vi "fpga_main.vi"() -> ()   [LabVIEW 2025]
uses:
  <vilib>/rvi/Emulation/niFpgaGetClockAttributes.vi
  <vilib>/rvi/Emulation/niFpgaSctlEmulationGetInTimedLoop.vi
  <vilib>/rvi/Emulation/niFpgaEmulationReportErrorSimple.vi
  <vilib>/rvi/Emulation/niFpgaEmulationIsFPGAContextNoSignature.vi
  <vilib>/rvi/errors/niFpgaSetErrorForExecOnDevCompSimple.vi
  <vilib>/rvi/eio/common/nirviEmuReportErrorAndStop.vi
  <vilib>/rvi/DataTransferAndStorage/Container/Common/niFpgaContainerGetUniqueNameForEmu.vi
  <vilib>/rvi/FIFO/Fifo_Resource/nirvififoEmulationSetSize.vi
  <vilib>/rvi/FIFO/Fifo_Resource/nirviFifoEmulationQueueMgr.vi
  <instcachedir>/0/nirviFifoEmulationQueueMgr_E5CAEC123FF24DC58D834DCA3CDAA9B5.lvgen/nirviFifoEmulationQueueMgr_E5CAEC123FF24DC58D834DCA3CDAA9B5_001.vi
  <vilib>/Utility/error.llb/Clear Errors.vi
  <vilib>/rvi/FIFO/Fifo_Resource/nirvififoEmulationCreateLock.vi
  <vilib>/rvi/Emulation/niFpgaProcessEmulError.vi
  <vilib>/rvi/FIFO/Fifo_Resource/nirvififoEmulationObtainLock.vi
  <vilib>/rvi/FIFO/Fifo_Resource/nirvififoEmulationReleaseLock.vi
  <vilib>/rvi/occurrence/nirviWaitOnOccurrenceBase.vi
  <vilib>/rvi/errors/nirviReportUnexpectedCaseInternalError.vi
  <vilib>/rvi/errors/nirviReportUnexpectedCaseInternalError (U32).vi
  <vilib>/eio/utilities/niEioResolveVilibRelativePath.vi
  <vilib>/rvi/interface/RandomDataEmulation/niFpgaRandomDataHandleErrors.vi
  <vilib>/rvi/Emulation/niFpgaCriticalErrorInLSC.vi
  <vilib>/rvi/eio/common/nirviEmuTemplateMethod_errors.vi
  <vilib>/rvi/Memory/Memory_Emulation/nirvimemoryFastEmulation.vi
  <vilib>/rvi/Memory/Memory_Emulation/nirvimemoryEmulation.vi
  <vilib>/rvi/FIFO/Fifo_Resource/nirvififoEmulationDetermineInputValidOut.vi
  <vilib>/rvi/DataTransferAndStorage/Container/XNode/niFpgaContainer.xnode
  <vilib>/rvi/FIFO/Fifo_Resource/nirvififoEmulationRead.vi
  <vilib>/rvi/interface/RandomDataEmulation/nirviRandomDataFpgaReadWriteTemplate.vi
  <vilib>/eio/EIONode/EIONode.xnode
  <vilib>/rvi/FIFO/Fifo_Resource/nirvififoEmulationWrite.vi
panel:
  in  "Var data":cluster{"Placeholder":i16, "Trigger":bool}
  in  "Time delay_Send":u16=1250
  in  "Time Delay_Read":u16=1250
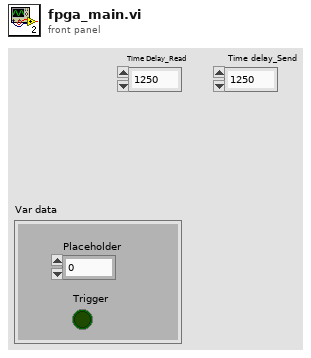
[diagram p1: front panel]
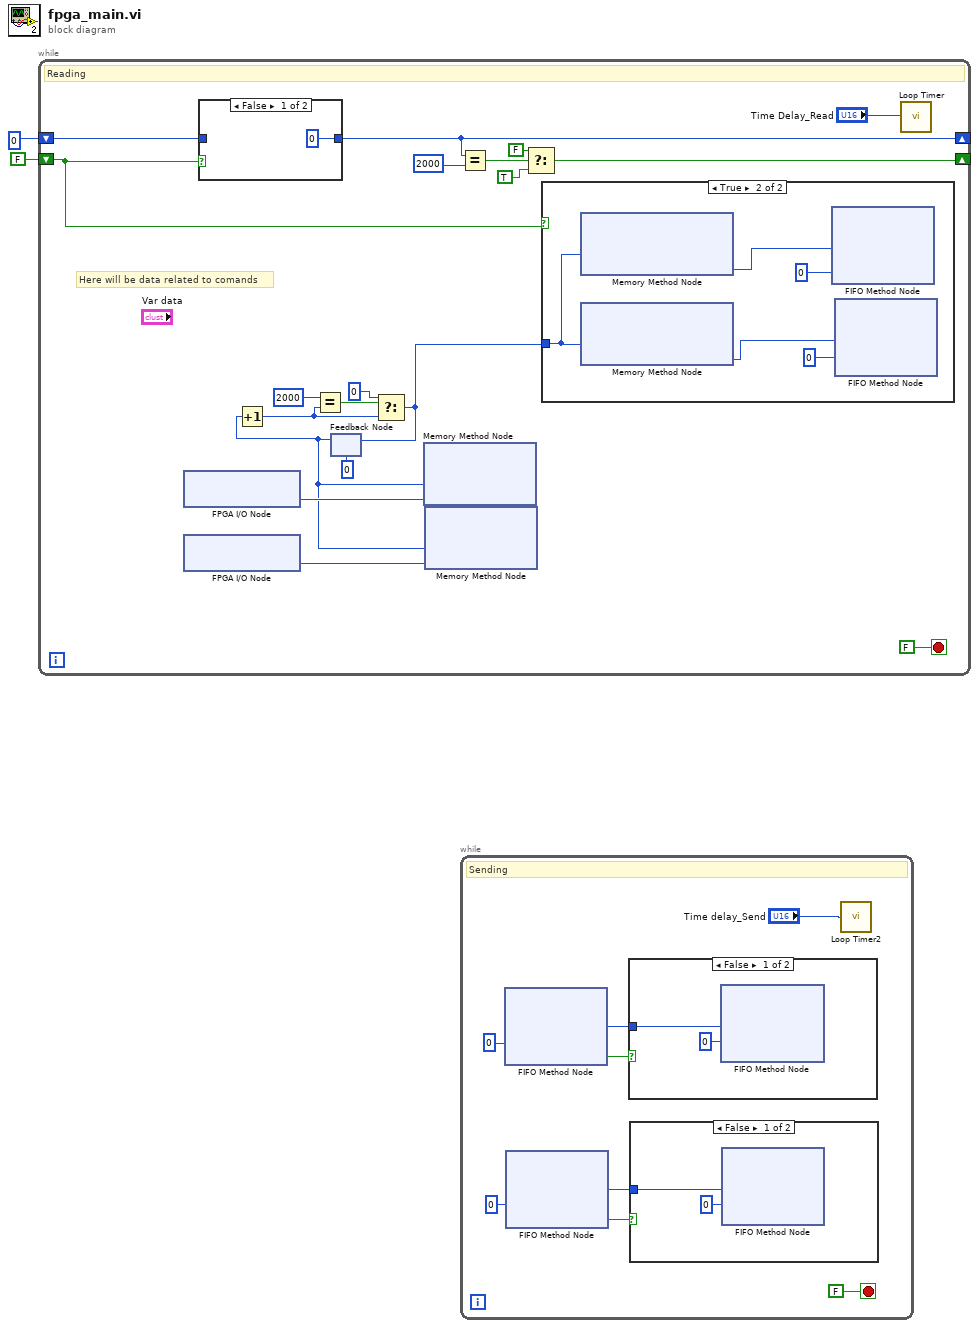
[diagram p0: block diagram]
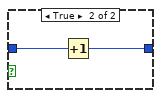
[diagram p4: hidden frame]
diagram:
  n1 = while {
    shift-right: [w11] -> _
    shift-left: FALSE ("t") -> [w4]
    shift-right: [w7] -> _
    shift-left: 0 ("Timeout") -> [w10]
    stop <- FALSE stop-if-true
    # "Here will be data related to comands"
    # "Reading"
    n2 = xnode "FPGA I/O Node"() -> ("AccelerationX"=w19:i16)  [unwired: 1 in, 1 out]
    n3 = xnode "FPGA I/O Node"() -> ("AccelerationY"=w14:i16)  [unwired: 1 in, 1 out]
    n4 = case shown="False" w4 {
      tunnel: [0 w24] -> w7
      tunnel: w10 -> [_ w23]
      frame False {
      }
      frame True {
        n5 = Increment(x=w23) -> (x+1=w24:i32)
      }
    }
    n6 = feedback #1(u32 0 ("Timeout")) -> (w13:u32)
    n7 = Increment(x=w13) -> (x+1=w15:u32)
    n8 = Equal?(x=u32 2000, y=w15) -> (x = y?=w17:bool)
    n9 = Select(t=u32 0, s=w17, f=w15) -> (s? t:f=w6:u32)
    n10 = feedback-in #1(w6) -> ()
    n11 = xnode ("Memory Method Node")("Address"=w13, "Data"=w19) -> ()  [unwired: 1 in, 1 out]
    n12 = xnode ("Memory Method Node")("Address"=w13, "Data"=w14) -> ()  [unwired: 1 in, 1 out]
    n13 = Equal?(x=w7, y=2000) -> (x = y?=w8:bool)
    n14 = Select(t=FALSE, s=w8, f=TRUE) -> (s? t:f=w11:bool)
    n15 = case shown="True" w4 {
      tunnel: w6 -> [_ w25]
      frame False {
      }
      frame True {
        n16 = xnode ("Memory Method Node")("Address"=w25) -> ("Data"=w28:i16)  [unwired: 1 in, 1 out]
        n17 = xnode ("Memory Method Node")("Address"=w25) -> ("Data"=w26:i16)  [unwired: 1 in, 1 out]
        n18 = xnode ("FIFO Method Node")("Element"=w28, "Timeout"=0) -> ()  [unwired: 1 in, 2 out]
        n19 = xnode ("FIFO Method Node")("Element"=w26, "Timeout"=0) -> ()  [unwired: 1 in, 2 out]
      }
    }
    n20 = call "Loop Timer"("Count(uSec)"="Time Delay_Read") -> ()  [unwired: 1 out]
  }
  n21 = while {
    stop <- FALSE stop-if-true
    # "Sending"
    n22 = xnode ("FIFO Method Node")("Timeout"=0) -> ("Element"=w35:i16, "Timed Out?"=w37:bool)  [unwired: 1 in, 1 out]
    n23 = xnode ("FIFO Method Node")("Timeout"=0) -> ("Element"=w32:i16, "Timed Out?"=w33:bool)  [unwired: 1 in, 1 out]
    n24 = case shown="False" w37 {
      tunnel: w35 -> [w41 _]
      frame False {
        n25 = xnode ("FIFO Method Node")("Element"=w41, "Timeout"=0) -> ()  [unwired: 1 in, 2 out]
      }
      frame True {
      }
    }
    n26 = case shown="False" w33 {
      tunnel: w32 -> [w39 _]
      frame False {
        n27 = xnode ("FIFO Method Node")("Element"=w39, "Timeout"=0) -> ()  [unwired: 1 in, 2 out]
      }
      frame True {
      }
    }
    n28 = call "Loop Timer2"("Count(uSec)"="Time delay_Send") -> ()  [unwired: 1 out]
  }
